vi "计算相机1补偿量.vi"(8 "取料对刀/复锁对刀":enum16{"取料补偿", "复锁补偿"}(ring), 9 "到校准时位置":enum16{"到校准时位置", "到画面中心"}(ring), 10 "取像时间":u32, 11 "Image In":T2) -> (0 "拍照结果":bool=TRUE, 1 "发送给PLC数据数组XYZR*1000+拧紧程式序号":dbl[](array[numeric]), 2 "视觉补偿机械手移动量mm":T5 {"X" format="%#.3f"}, 3 "Image":T2(plugin-control), 4 "存档数据和结果 out":T4={"待写入数据"=[], "单个结果"=[], "总结果"=FALSE, "数据有效"=TRUE})   [LabVIEW 2014]
uses:
  Global.vi
  Controls/XYPos.ctl
  Controls/TestThreshold.ctl
  <vilib>/vision/Image Controls.llb/IMAQ Image.ctl
panel:
  out "机械手移动量XY mm+螺丝刀旋转角度在规格内数组":bool[](array[boolean])
  in  "30量测规格数组 in":T1[](array[typedef])=[{"下限"=1.8, "上限"=2.2}, {"下限"=0.7, "上限"=1.2}, {"下限"=0.0, "上限"=8.0}, {"下限"=0.0, "上限"=8.0}] {"上限" format="%#.4g"; "下限" format="%#.4g"}
  in  "25量测规格数组 in":T1[](array[typedef])=[{"下限"=1.6, "上限"=2.0}, {"下限"=0.8, "上限"=1.25}, {"下限"=0.0, "上限"=8.0}, {"下限"=0.0, "上限"=8.0}] {"上限" format="%#.4g"; "下限" format="%#.4g"}
  out "螺帽内径mm":dbl
  in  "选项卡控件":enum32{"选项卡 1", "选项卡 2"}(tab)
  out "Fitted Circle":T3 {"Average SNR (dB)" format="%.2f"; "Average Strength" format="%.2f"; "Roundness (Real-World)" format="%.2f"; "Radius (Real-World)" format="%.2f"; "Center (Real-World)"."Y" format="%.2f"; "Center (Real-World)"."X" format="%.2f"; "Radius (Pixels)" format="%.2f"; "Center (Pixels)"."Y" format="%.2f"; "Center (Pixels)"."X" format="%.2f"}
  out "定位圆找-螺帽内径在规格内":bool
  out "一字槽中心":cluster{"X":sgl, "Y":sgl}
  in  "量测项目名称":string[](array[string])=["一字槽位置偏移量X(mm)", "一字槽位置偏移量Y(mm)", "一字槽角度(度)", "螺丝刀要旋转角度(度)", ""]
  in  "显示内容名称":string[](array[string])=["螺帽内径(mm)", "一字槽宽度(mm)", "一字槽两边角度差异(度)", "一字槽两边与缺口连线角度差异(度)"]
  out "螺帽中心":cluster{"X Centroid":sgl, "Y Centroid":sgl} {"Y Centroid" format="%.2f"; "X Centroid" format="%.2f"}
  out "拧紧程式序号数组":i32[](array[numeric])
  out "一字槽角度":dbl
  out "图像信息结果":bool[](array[boolean])
  out "图像信息":dbl[](array[numeric])
  out "视觉补偿mm+槽角度+螺丝刀旋转角度":dbl[](array[numeric])
  out "视觉补偿量合理":bool
  in  "ImgPath":path=path "E:/771/771半自动装配系统-20200818/校准/上相机拍照-螺丝刀原点时-对位完成后拍照螺丝槽.jpg"
  # "~"
  # "~"
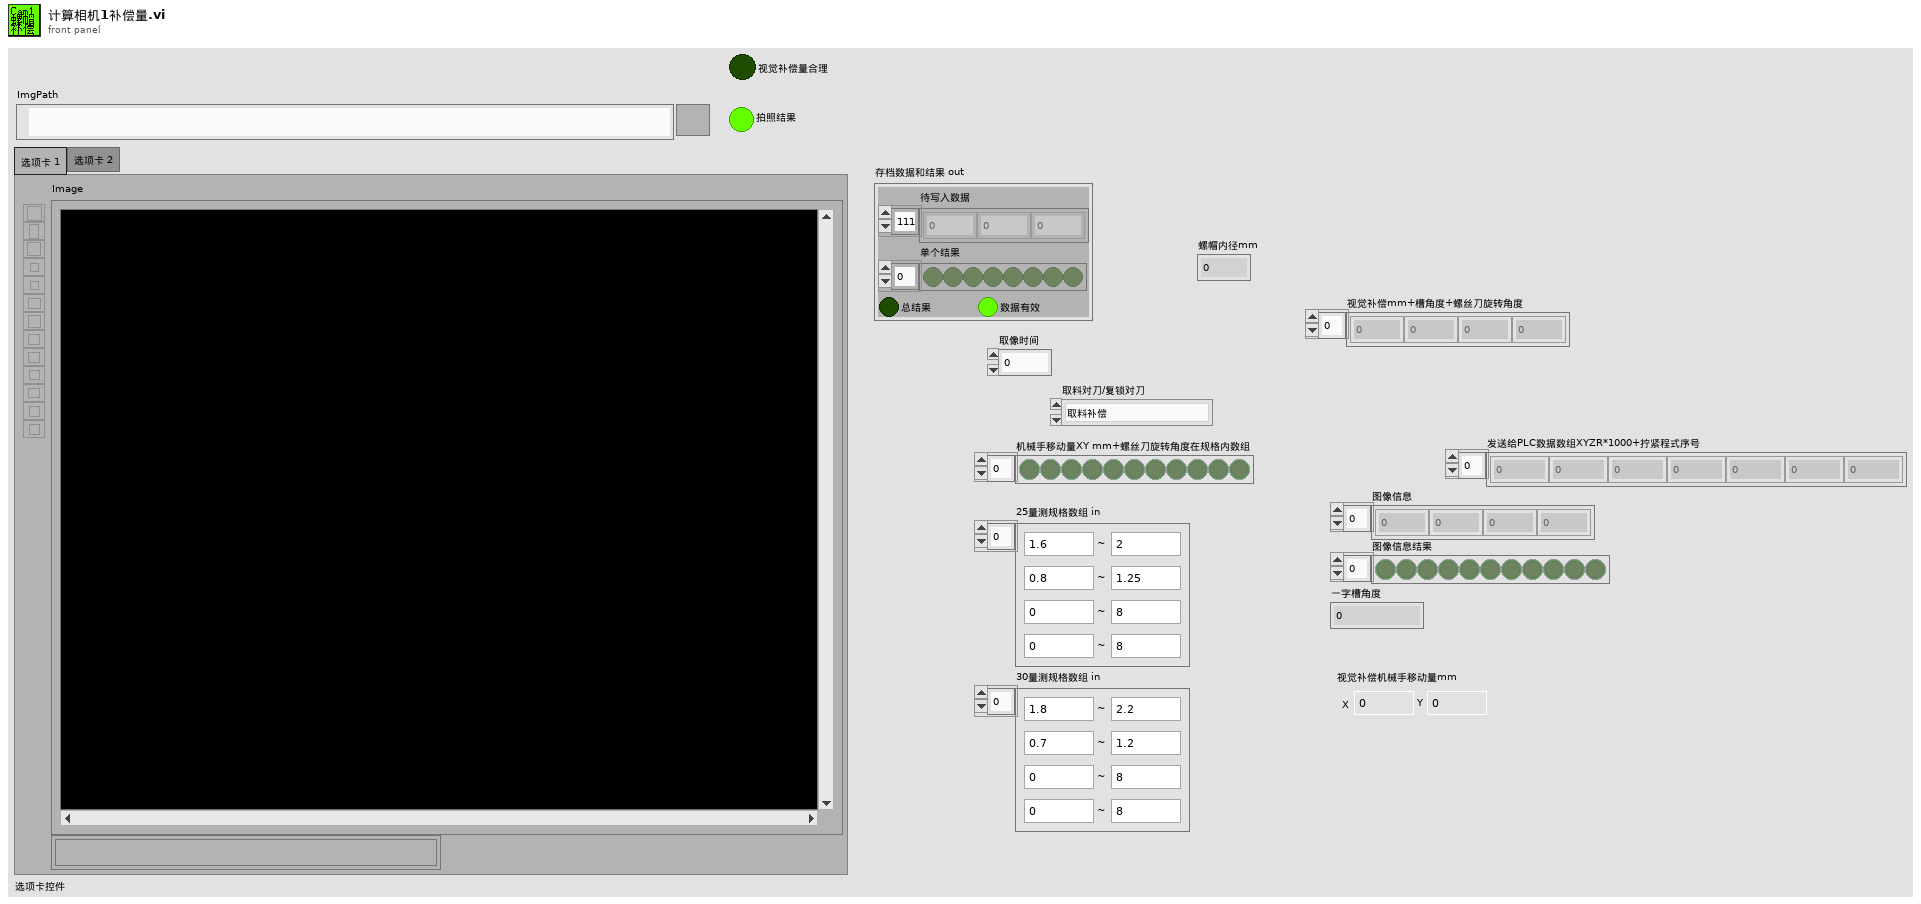
[diagram p1: front panel]
types:
  T1 = typedef "TestThreshold.ctl" = cluster{"下限":dbl, "上限":dbl}
  T2 = typedef "IMAQ Image.ctl" = refnum<image>
  T3 = cluster{"Center (Pixels)":cluster{"X":sgl, "Y":sgl}, "Radius (Pixels)":dbl, "Center (Real-World)":cluster{"X":sgl, "Y":sgl}, "Radius (Real-World)":dbl, "Roundness (Real-World)":dbl, "Average Strength":dbl, "Average SNR (dB)":dbl}
  T4 = typedef "存档数据和结果.ctl" = cluster{"待写入数据":dbl[], "单个结果":bool[], "总结果":bool, "数据有效":bool}
  T5 = typedef "XYPos.ctl" = cluster{"X":dbl, "Y":dbl}
  T6 = typedef "欧姆龙PLC Action.ctl" = enum16{"读设备状态", "初始化", "待命", "重新初始化", "读触发信息", "读第1组Mark点坐标", "读第2组Mark点坐标", "写基本信息", "写第1组Mark点坐标", "写第2组Mark点坐标", "写相机中心到出线头的距离", "写一笔轨迹到PLC", "写入进线前段点位", "写入板内布线点位", "写入出线布线点位", "写入数据写入完成信号", "获取信息", "写入进出线方向", "写加工信号"}
  T7 = typedef "ModeEditeControl.ctl" = cluster{"AllModelFold":path, "AllModelNamePath":path, "所有零件型号":string[], "当前零件型号":string, "所有建立零件信息":string[][], "当前零件序号":i32, "当前产品信息":T8}
  T8 = typedef "ModelInfo.ctl" = cluster{"产品型号":string, "二维码拍照":u32, "Mark点拍照":u32}
  T9 = typedef "OtherSpec.ctl" = cluster{"其它勾选类规格":T10, "其它数据类规格":T11, "相机名称":T12, "参数":cluster{"Mark1曝光时间":i32, "Mark2曝光时间":i32, "二维码曝光时间":i32}}
  T10 = typedef "其它勾选类规格.ctl" = cluster{"保存图片":bool, "上传设备状态数据":bool, "保存数据":bool, "开机默认开启监控摄像头":bool, "启用mark拍照 ":bool}
  T11 = typedef "其他数据类规格.ctl" = cluster{"相机1像素-毫米换算系数":dbl, "相机2像素-毫米换算系数":dbl, "D盘剩余空间预警(G)":dbl, "视频最长录制时间(秒)":dbl}
  T12 = typedef "相机名称品牌使用状态.ctl" = cluster{"相机1名称":T13, "相机2名称":T13, "Cam1启用":bool, "Cam2启用":bool, "Basler1":bool, "Basler2":bool}
  T13 = typedef "IMAQdx.ctl" = refnum<k21>
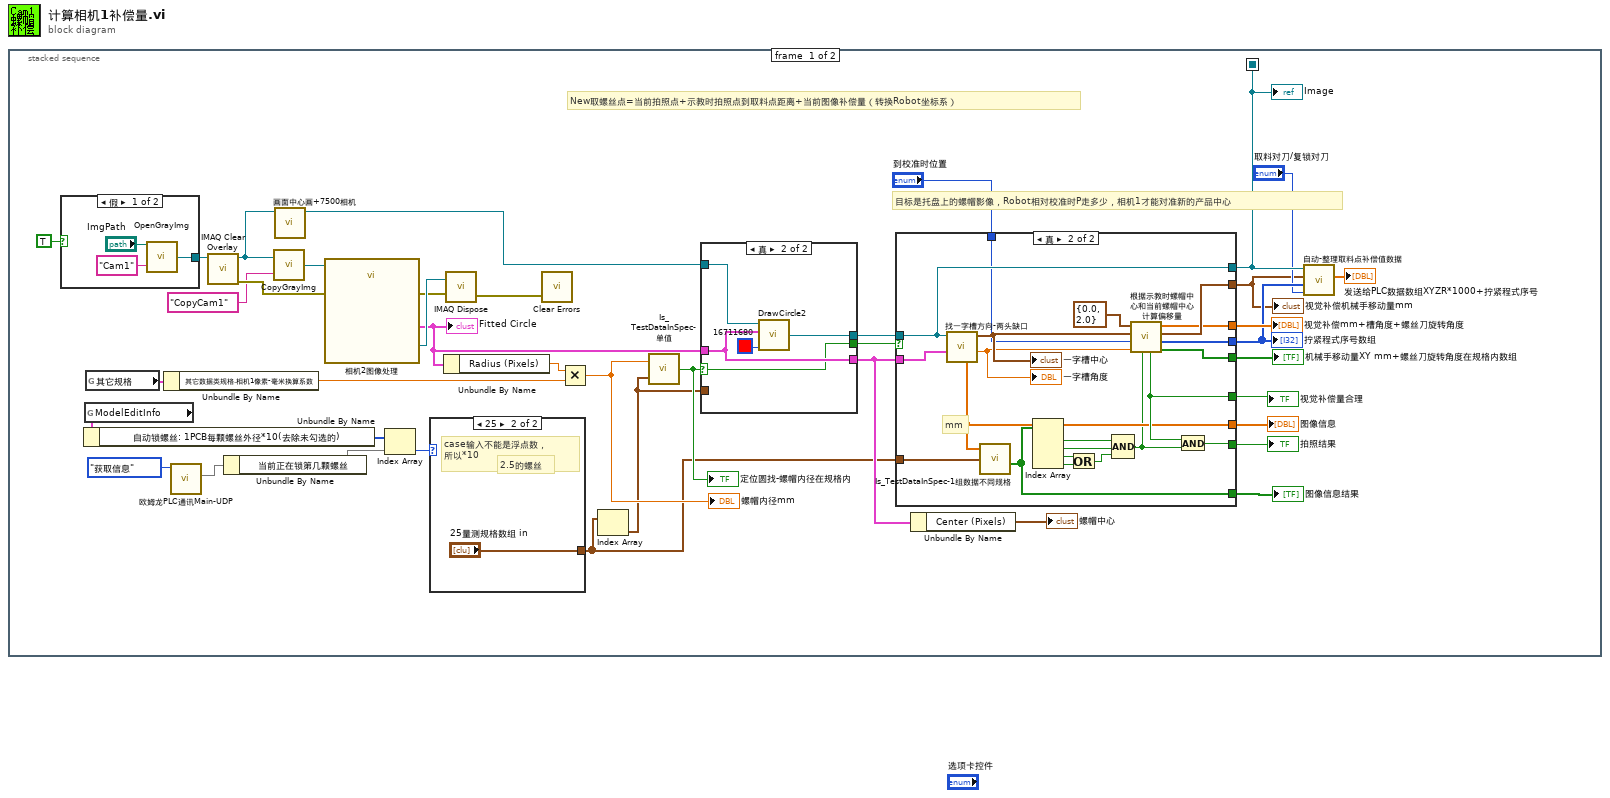
[diagram p0: block diagram]
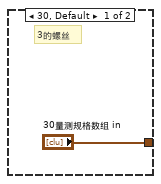
[diagram p2: hidden frame]
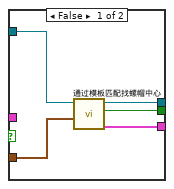
[diagram p3: hidden frame]
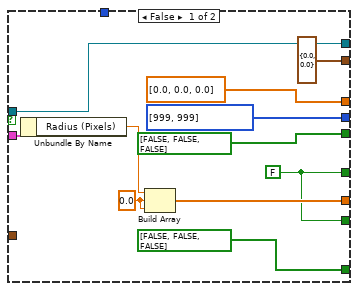
[diagram p4: hidden frame]
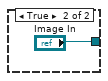
[diagram p5: hidden frame]
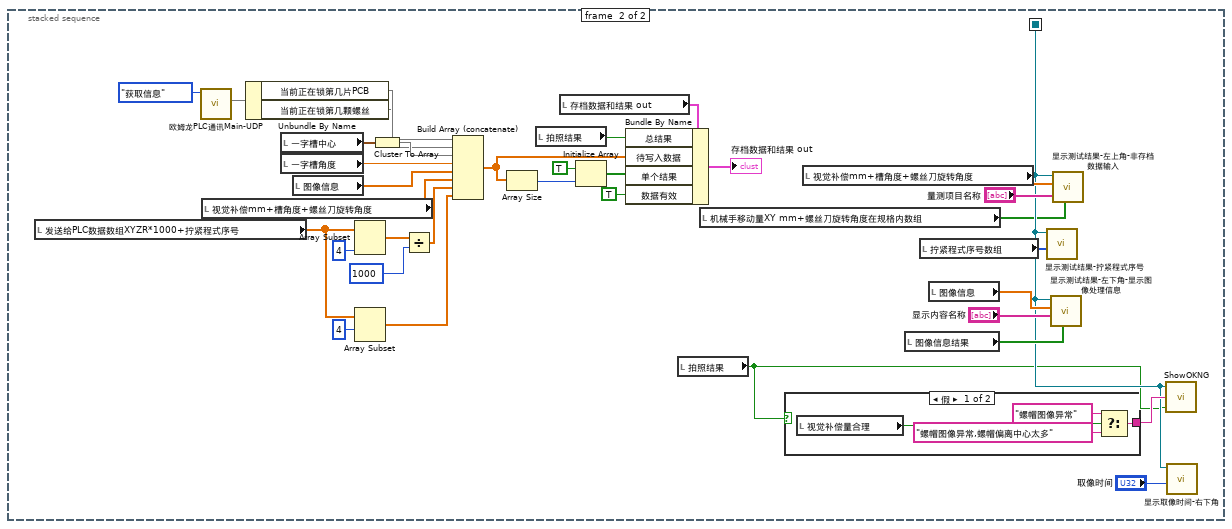
[diagram p6: hidden frame]
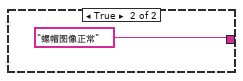
[diagram p7: hidden frame]
diagram:
  n1 = stacked-sequence {
    seq-local: [w20 _] -> [_ w115]
    frame #0 {
      # "New取螺丝点=当前拍照点+示教时拍照点到取料点距离+当前图像补偿量（转换Robot坐标系）"
      # "目标是托盘上的螺帽影像，Robot相对校准时P走多少，相机1才能对准新的产品中心"
      n2 = case shown="假" TRUE {
        tunnel: [w86 "Image In"] -> w33
        frame False {
          n3 = call "OpenGrayImg.vi"("Image Name"="Cam1", "Img Path"="ImgPath") -> ("Image Out"=w86:T2)
        }
        frame True {
        }
      }
      n4 = global read "Global.vi" "ModelEditInfo"() -> (w13:T7)
      n5 = Unbundle By Name(w13) -> ("自动锁螺丝: 1PCB每颗螺丝外径*10(去除未勾选的)"=w12:u32[])
      n6 = global read "Global.vi" "其它规格"() -> (w9:T9)
      n7 = Unbundle By Name(w9) -> ("其它数据类规格.相机1像素-毫米换算系数"=w5:dbl)
      n8 = call "欧姆龙PLC通讯Main-UDP.vi"("欧姆龙PLC Action"=欧姆龙PLC_Action."获取信息") -> (2:w14)  [unwired: 7 in, 3 out]
      n9 = call "IMAQ Clear Overlay"("Image"=w33) -> ("error out"=w40:errorcluster, "Image Out"=w25:T2)  [unwired: 9 in]
      n10 = Unbundle By Name(w14) -> ("当前正在锁第几颗螺丝"=w11)
      n11 = call "CopyGrayImg.vi"("Image Name"="CopyCam1", "Image In"=w25) -> ("Image Out"=w31:T2)
      n12 = call "画面中心画+7500相机.vi"("引用句柄输入"=w25) -> ("引用句柄输出"=w24:T2)  [unwired: 10 in]
      n13 = call "相机2图像处理"("Image In"=w31, "error in"=w40) -> ("Image Out"=w30:T2, "Fitted Circle (Find Circular Edge 1)"=w6:T3, "error out"=w29:errorcluster)  [unwired: 23 in]
      "Fitted Circle" <- w6
      n14 = Index Array(array=w12, index=w11) -> (element=w10:u32)
      n15 = case shown="25" w10 {
        tunnel: ["30量测规格数组 in" "25量测规格数组 in"] -> w2
        frame 30, Default {
          # "3的螺丝"
        }
        frame 25 {
          # "2.5的螺丝"
          # "case输入不能是浮点数，\n所以*10"
        }
      }
      n16 = Unbundle By Name(w6) -> ("Radius (Pixels)"=w8:dbl)
      n17 = call "IMAQ Dispose"("Image"=w30, "error in (no error)"=w29) -> ("error out"=w26:errorcluster)  [unwired: 4 in]
      n18 = call <vilib>:"Clear Errors.vi"("error in (no error)"=w26) -> ()  [unwired: 5 in, 2 out]
      n19 = Multiply(x=w8, y=w5) -> (x*y=w7:dbl)
      "螺帽内径mm" <- w7
      n20 = Index Array(array=w2) -> (element=w1:T1)  [unwired: 1 in]
      n21 = call "Is_TestDataInSpec-单值.vi"("量测规格"=w1, "相机量测结果"=w7) -> ("在规格内"=w27:bool)
      "定位圆找-螺帽内径在规格内" <- w27
      n22 = case shown="真" w27 {
        selector: w27 -> [_ w49]
        tunnel: w6 -> [_ w51]
        tunnel: [w45 w51] -> w28
        tunnel: [w43 w50] -> w35
        tunnel: [w47 w49] -> w34
        tunnel: w24 -> [w44 w48]
        tunnel: w1 -> [w46 _]
        frame False {
          n23 = call "通过模板匹配找螺帽中心.vi"("量测规格"=w46, "Img输入"=w44) -> ("Fitted Circle"=w45:T3, "在规格内"=w47:bool, "Img输入 out"=w43:T2)  [unwired: 6 in, 1 out]
        }
        frame True {
          n24 = call "DrawCircle2.vi"("Color"=u32 16711680, "Fitted Circle (左圆)"=w51, "Img in"=w48) -> ("Img out"=w50:T2)  [unwired: 1 in]
        }
      }
      n25 = case shown="真" w34 {
        tunnel: w35 -> [w61 w83]
        tunnel: [dbl[] [0.0, 0.0, 0.0] w76] -> w38
        tunnel: [i32[] [999, 999] ("拧紧程式序号数组") w75] -> w19
        tunnel: w28 -> [w54 w84]
        tunnel: [w61 w83] -> w20
        tunnel: [w60 w71] -> w22
        tunnel: [w56 w81] -> w36
        tunnel: [bool[] [FALSE, FALSE, FALSE] w70] -> w21
        tunnel: [w56 w74] -> w23
        tunnel: [T5 {"X"=0.0, "Y"=0.0} ("机械手移动量 mm") w80] -> w16
        tunnel: w2 -> [_ w79]
        tunnel: "到校准时位置" -> [_ w78]
        tunnel: [bool[] [FALSE, FALSE, FALSE] ("机械手移动量XY mm+螺丝刀旋转角度在规格内数组") w73] -> w3
        frame False {
          w56 = FALSE
          w59 = 0.0 ("元素")
          n26 = Unbundle By Name(w54) -> ("Radius (Pixels)"=w53:dbl)
          n27 = Build Array(w53, w59, w59) -> (w60:dbl[])
        }
        frame True {
          # "mm"
          n28 = call "找一字槽方向-两头缺口.vi"("Fitted Circle"=w84, "Img in"=w83) -> ("一字槽角度"=w77:dbl, "一字槽中心"=w82:cluster{"X":sgl, "Y":sgl}, "半径+槽宽+角度差异mm"=w71:dbl[])  [unwired: 7 in]
          "一字槽中心" <- w82
          "一字槽角度" <- w77
          n29 = call "Is_TestDataInSpec-1组数据不同规格.vi"("相机量测结果"=w71, "量测规格数组 in"=w79) -> ("数组"=w70:bool[])  [unwired: 2 in, 2 out]
          n30 = Index Array(array=w70) -> (element #1=w69:bool, element #2=w68:bool, element #3=w67:bool, element #4=w66:bool)  [unwired: 4 in]
          n31 = Or(x=w67, y=w66) -> (x .or. y?=w65:bool)
          n32 = Compound Arithmetic op=AND(w69, w68, w65) -> (w64:bool)
          n33 = call "根据示教时螺帽中心和当前螺帽中心计算偏移量.vi"("半径槽宽角度正常"=w64, "一字槽角度"=w77, "到校准时位置"=w78, "一字槽中心"=w82, "一字槽中心允许偏移量"=T1 {"下限"=0.0, "上限"=2.0}) -> ("机械手移动量XY mm+螺丝刀旋转角度在规格内数组"=w73:bool[], "拧紧程式序号数组"=w75:i32[], "机械手移动量 mm"=w80:T5, "机械手移动量XY mm+槽角度+螺丝刀旋转角度"=w76:dbl[], "一字槽中心偏移量在规格内"=w74:bool)  [unwired: 2 in]
          n34 = And(x=w74, y=w64) -> (x .and. y?=w81:bool)
        }
      }
      "Image" <- w20
      "拧紧程式序号数组" <- w19
      "拍照结果" <- w36
      "视觉补偿量合理" <- w23
      "视觉补偿mm+槽角度+螺丝刀旋转角度" <- w38
      "图像信息" <- w22
      "图像信息结果" <- w21
      "视觉补偿机械手移动量mm" <- w16
      "机械手移动量XY mm+螺丝刀旋转角度在规格内数组" <- w3
      n35 = Unbundle By Name(w28) -> ("Center (Pixels)"=→"螺帽中心":cluster{"X":sgl, "Y":sgl})
      n36 = call "自动-整理取料点补偿值数据.vi"("取料对刀/复锁对刀"="取料对刀/复锁对刀", "拧紧程式序号数组"=w19, "上视觉补偿机械手移动量 mm输入"=w16, "Img输入"=w20) -> ("发送给PLC数据数组"=→"发送给PLC数据数组XYZR*1000+拧紧程式序号":dbl[])  [unwired: 6 in, 1 out]
    }
    frame #1 {
      n37 = local read "发送给PLC数据数组XYZR*1000+拧紧程式序号"() -> (w93:dbl[])
      n38 = call "欧姆龙PLC通讯Main-UDP.vi"("欧姆龙PLC Action"=欧姆龙PLC_Action."获取信息") -> (2:w100)  [unwired: 7 in, 3 out]
      n39 = local read "视觉补偿mm+槽角度+螺丝刀旋转角度"() -> (w110:dbl[])
      n40 = Unbundle By Name(w100) -> ("当前正在锁第几片PCB"=w99, "当前正在锁第几颗螺丝"=w98)
      n41 = local read "一字槽中心"() -> (w114:cluster{"X":sgl, "Y":sgl})
      n42 = local read "一字槽角度"() -> (w111:dbl)
      n43 = local read "图像信息"() -> (w112:dbl[])
      n44 = Array Subset(array=w93, length=4 ("长度")) -> (w96:dbl[])  [unwired: 1 in]
      n45 = Array Subset(array=w93, index=4 ("索引")) -> (w91:dbl[])  [unwired: 1 in]
      n46 = Cluster To Array(cluster=w114) -> (array=w113:sgl[])
      n47 = Divide(x=w96, y=1000 ("元素")) -> (x/y=w95:dbl[])
      n48 = Build Array (concatenate)(w99, w98, w113, w111, w112, w110, w95, w91) -> (w103:dbl[])
      n49 = Array Size(array=w103) -> (size(s)=w106:i32)
      n50 = local read "拍照结果"() -> (w102:bool)
      n51 = local read "存档数据和结果 out"() -> (w104:T4)
      n52 = Initialize Array(TRUE, w106) -> (w107:bool[])
      n53 = Bundle By Name(cluster=w104, "总结果"=w102, "待写入数据"=w103, "单个结果"=w107, "数据有效"=TRUE) -> (→"存档数据和结果 out":T4)
      n54 = local read "拍照结果"() -> (w90:bool)
      n55 = local read "机械手移动量XY mm+螺丝刀旋转角度在规格内数组"() -> (w89:bool[])
      n56 = case shown="假" w90 {
        tunnel: [w126 "螺帽图像正常" ("显示消息")] -> w121
        frame False {
          n57 = local read "视觉补偿量合理"() -> (w125:bool)
          n58 = Select(t="螺帽图像异常" ("显示消息"), s=w125, f="螺帽图像异常,螺帽偏离中心太多") -> (s? t:f=w126:string)
        }
        frame True {
        }
      }
      n59 = local read "视觉补偿mm+槽角度+螺丝刀旋转角度"() -> (w123:dbl[])
      n60 = local read "图像信息结果"() -> (w117:bool[])
      n61 = local read "拧紧程式序号数组"() -> (w120:i32[])
      n62 = local read "图像信息"() -> (w118:dbl[])
      n63 = call "显示测试结果-拧紧程式序号.vi"("拧紧程式序号数组"=w120, "Img输入"=w115) -> ()  [unwired: 10 in]
      n64 = call "显示测试结果-左下角-显示图像处理信息.vi"("每个数据结果"=w117, "量测项目名称"="显示内容名称", "显示数据"=w118, "Img输入"=w115) -> ()  [unwired: 8 in]
      n65 = call "显示测试结果-左上角-非存档数据输入.vi"("单个数据结果"=w89, "量测项目名称"="量测项目名称", "显示数据"=w123, "Img输入"=w115) -> ()  [unwired: 7 in, 1 out]
      n66 = call "ShowOKNG.vi"("结果"=w90, "显示消息"=w121, "引用句柄输入"=w115) -> ()
      n67 = call "显示取像时间-右下角.vi"("取像时间"="取像时间", "引用句柄输入"=w115) -> ()  [unwired: 9 in, 1 out]
    }
  }
